vi "3_data_type_2.vi"() -> ()   [LabVIEW 2015]
panel:
  in  "열거형":enum16{""}(ring)
  out "출력 클러스터":cluster{"번호":i32, "운영시간":bool, "이름":string}
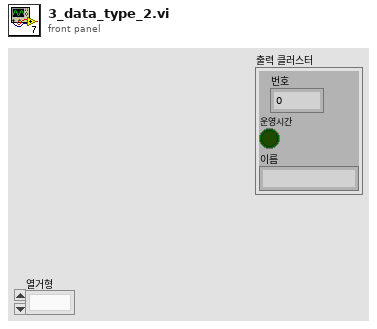
[diagram p1: front panel]
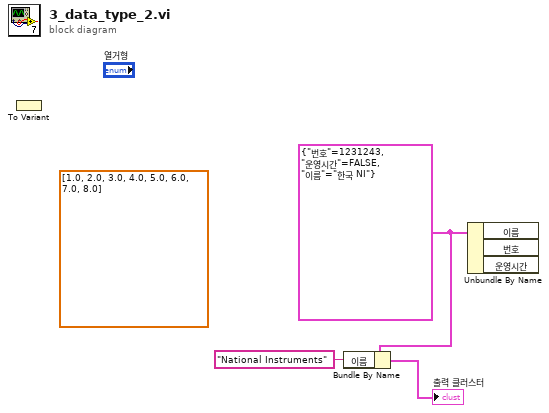
[diagram p0: block diagram]
diagram:
  w3 = cluster{"번호":i32, "운영시간":bool, "이름":string} {"번호"=1231243, "운영시간"=FALSE, "이름"="한국 NI"}
  (unwired) dbl[][] [[1.0, 2.0, 3.0, 4.0, 5.0, 6.0, 7.0, 8.0]]
  n1 = To Variant() -> ()  [unwired: 1 in, 1 out]
  n2 = Bundle By Name(cluster=w3, "이름"="National Instruments") -> (→"출력 클러스터":cluster{"번호":i32, "운영시간":bool, "이름":string})
  n3 = Unbundle By Name(w3) -> ()  [unwired: 3 out]
